vi "Display QDFunction Info In QuickBox.vi"(8 "error in (no error)":errorcluster, 11 "QDFunction in":refnum<class "QDFunction.lvclass">) -> (0 "error out":errorcluster, 2 "Content For Display":string, 3 "QDFunction out":refnum<class "QDFunction.lvclass">)   [LabVIEW 2015, in "QDFunction.lvclass"]
uses:
  QDFunction.lvclass
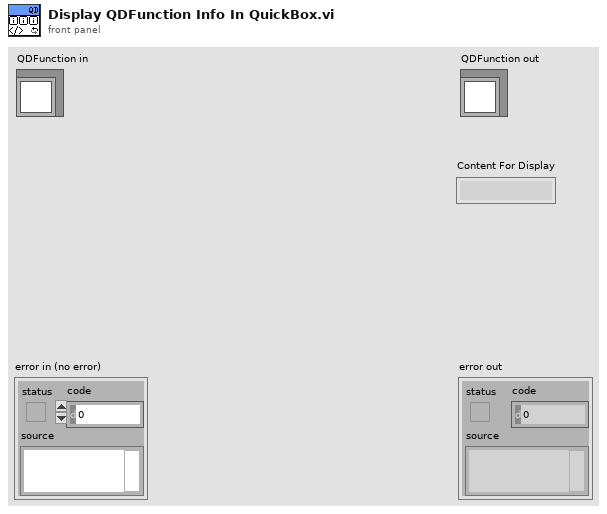
[diagram p1: front panel]
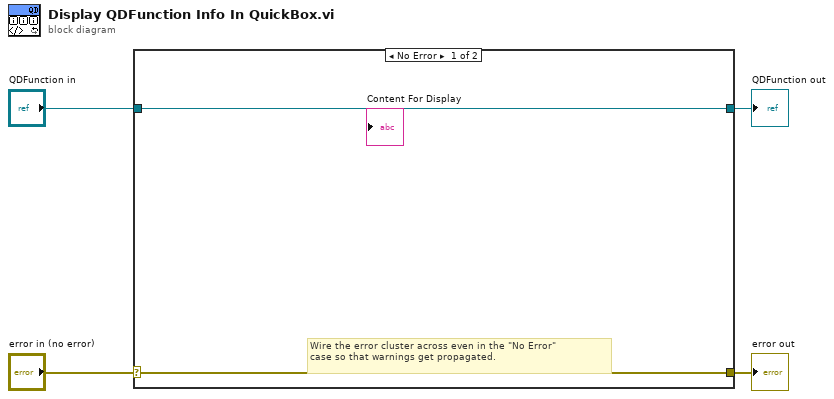
[diagram p0: block diagram]
diagram:
  n1 = case shown="No Error" "error in (no error)" {
    selector: "error in (no error)" -> [w5 w8]
    tunnel: [w5 w8] -> w3
    tunnel: [w6 w7] -> w1
    tunnel: "QDFunction in" -> [w6 w7]
    frame No Error {
      # "Wire the error cluster across even in the \"No Error\"\ncase so that warnings get propagated."
    }
    frame Error {
    }
  }
  "error out" <- w3
  "QDFunction out" <- w1
